vi "Write UI References.vi"(8 "error in (no error)":errorcluster, 10 "UI References":T1, 11 "UI Console in":refnum<class "UI Console.lvclass">) -> (0 "error out":errorcluster, 3 "UI Console out":refnum<class "UI Console.lvclass">)   [LabVIEW 2019, in "UI Console.lvclass"]
uses:
  UI Console.lvclass
  TypeDef/UI References.ctl
  UI Console.lvclass/UI Console.ctl
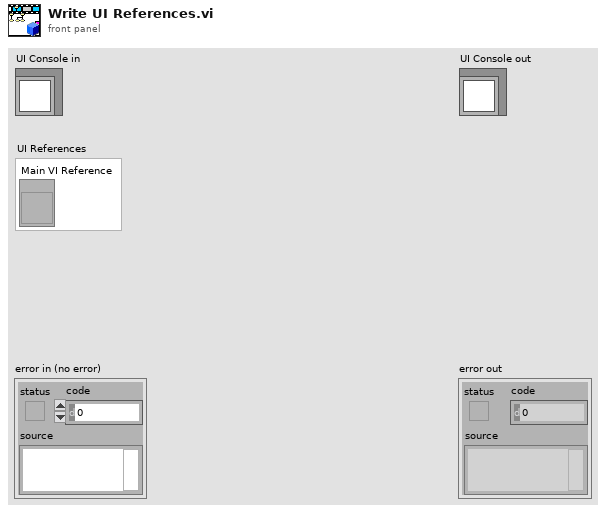
[diagram p1: front panel]
types:
  T1 = typedef "UI References.ctl" = cluster{"Main VI Reference":refnum<vi>}
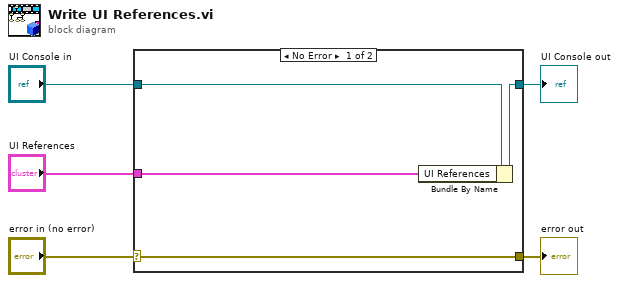
[diagram p0: block diagram]
diagram:
  n1 = case shown="No Error" "error in (no error)" {
    selector: "error in (no error)" -> [w9 w10]
    tunnel: [w9 w10] -> w4
    tunnel: [w7 w11] -> w2
    tunnel: "UI Console in" -> [w8 w11]
    tunnel: "UI References" -> [w6 _]
    frame No Error {
      n2 = Bundle By Name(cluster=w8, "UI References"=w6) -> (w7:refnum<class "UI Console.lvclass">)
    }
    frame Error {
    }
  }
  "error out" <- w4
  "UI Console out" <- w2
